vi "write_pulse.vi"(6 "Enum":T1(ring), 7 "error in":errorcluster, 8 "data":u8, 9 "lines":tag) -> (0 "error out":errorcluster)   [LabVIEW 2015]
uses:
  <vilib>/DAQmx/write.llb/DAQmx Write (Digital U8 1Chan 1Samp).vi
  <vilib>/DAQmx/create/channels.llb/DAQmx Create Channel (DO-Digital Output).vi
  <vilib>/DAQmx/configure/timing.llb/DAQmx Timing (Sample Clock).vi
  <vilib>/DAQmx/miscellaneous.llb/DAQmx Fill In Error Info.vi
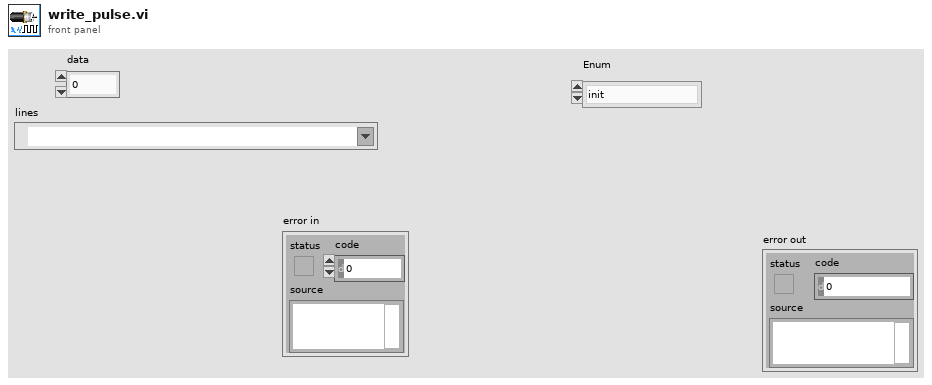
[diagram p1: front panel]
types:
  T1 = enum16{"init", "config", "start", "write", "stop"}
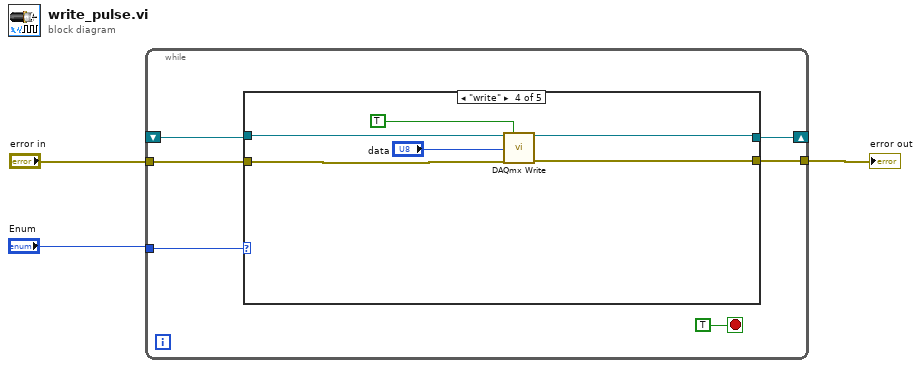
[diagram p0: block diagram]
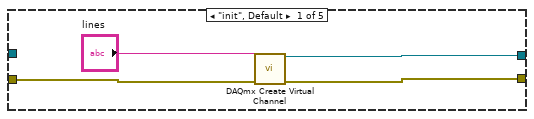
[diagram p2: hidden frame]
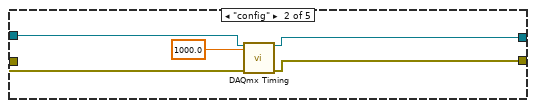
[diagram p3: hidden frame]
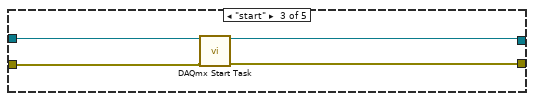
[diagram p4: hidden frame]
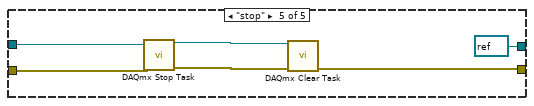
[diagram p5: hidden frame]
diagram:
  n1 = while {
    tunnel: "Enum" -> [w8]
    shift-right: [w7] -> _
    shift-left: _ -> [w6]
    tunnel: "error in" -> [w5]
    tunnel: [w4] -> w1
    stop <- TRUE stop-if-true
    n2 = case shown="\"write\"" w8 {
      tunnel: [w12 w16 w21 w27 refnum<k21> refnum ("task out")] -> w7
      tunnel: w6 -> [_ w17 w22 w28 w33]
      tunnel: w5 -> [w13 w18 w20 w23 w32]
      tunnel: [w11 w15 w19 w26 w30] -> w4
      frame "init", Default {
        n3 = call-poly <vilib>:"DAQmx Create Virtual Channel.vi"("lines"="lines", "error in"=w13) -> ("task out"=w12:refnum<k21>, "error out"=w11:errorcluster)  [unwired: 12 in]
      }
      frame "config" {
        n4 = call-poly <vilib>:"DAQmx Timing.vi"("task/channels in"=w17, "rate"=1000.0, "error in"=w18) -> ("task out"=w16:refnum<k21>, "error out"=w15:errorcluster)  [unwired: 11 in]
      }
      frame "start" {
        n5 = call <vilib>:"DAQmx Start Task.vi"("task/channels in"=w22, "error in"=w20) -> ("task out"=w21:refnum<k21>, "error out"=w19:errorcluster)  [unwired: 12 in]
      }
      frame "write" {
        n6 = call-poly <vilib>:"DAQmx Write.vi"("task/channels in"=w28, "auto start"=TRUE, "data"="data", "error in"=w23) -> ("task out"=w27:refnum<k21>, "error out"=w26:errorcluster)  [unwired: 9 in, 1 out]
      }
      frame "stop" {
        n7 = call <vilib>:"DAQmx Stop Task.vi"("task/channels in"=w33, "error in"=w32) -> ("task out"=w34:refnum<k21>, "error out"=w31:errorcluster)  [unwired: 12 in]
        n8 = call <vilib>:"DAQmx Clear Task.vi"("task in"=w34, "error in"=w31) -> ("error out"=w30:errorcluster)  [unwired: 13 in]
      }
    }
  }
  "error out" <- w1
